vi "Set the TimeInterval According to Range in Autosetup_FP-Scope SP.vi"(5 "Rate":dbl, 7 "Points":i32) -> (8 "VoltInterval":i32)   [LabVIEW 2012]
doc: "根据自动调整后采样率以及points获取timeinterval"
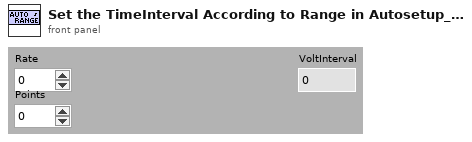
[diagram p1: front panel]
types:
  T1 = typedef "INI Properties_DStr-Scope SP.ctl" = cluster{"Channels":cluster{"String":string, "Value":ext}[], "VoltInterval":cluster{"String":string, "Value":ext}[], "Impedance":cluster{"String":string, "Value":ext}[], "Bandwidth":cluster{"String":string, "Value":ext}[], "TimeInterval":cluster{"String":string, "Value":ext}[], "Type":cluster{"String":string, "Value":ext}[], "Source":cluster{"String":string, "Value":ext}[], "DigiSource":cluster{"String":string, "Value":ext}[], "TrigCpl":cluster{"String":string, "Value":ext}[], "EXTCpl":cluster{"String":string, "Value":ext}[], "Mode":cluster{"String":string, "Value":ext}[], "Event":cluster{"String":string, "Value":ext}[], "Format":cluster{"String":string, "Value":ext}[], "OffsetVisible":bool[], "Offset":dbl[][], "Point":dbl[][], "TrigLev":dbl[][], "Win":dbl[][], "Leve":dbl[][], "ExtLev":dbl[][], "PolaEnable":u8, "RISEnable":u8, "ChanCpl":cluster{"String":string, "Value":ext}[], "TimeValue":dbl[], "VoltValue":dbl[], "ImpedanceValue":dbl[], "BandwidthValue":dbl[]}
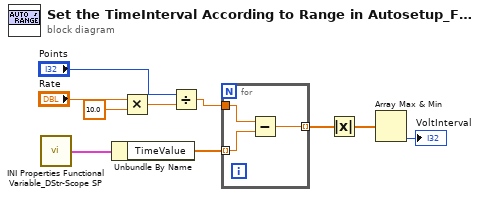
[diagram p0: block diagram]
diagram:
  n1 = call "INI Properties Functional Variable_DStr-Scope SP.vi"() -> ("proper"=w5:T1)  [unwired: 15 in]
  n2 = Unbundle By Name(w5) -> ("TimeValue"=w4:dbl[])
  n3 = Multiply(x="Rate", y=10.0 ("x")) -> (x*y=w2:dbl)
  n4 = Divide(x="Points", y=w2) -> (x/y=w1:dbl)
  n5 = for {
    tunnel: w4 -> [w12] mode=indexing
    tunnel: w1 -> [w13]
    tunnel: [w11] -> w8 mode=indexing
    n6 = Subtract(x=w13, y=w12) -> (x-y=w11:dbl)
  }
  n7 = Absolute Value(x=w8) -> (abs(x)=w7:dbl[])
  n8 = Array Max & Min(array=w7) -> (min index (indices)=→"VoltInterval":i32)  [unwired: 3 out]
